vi "To Start and Stop (bare).vi"(4 "span":dbl, 6 "center":dbl) -> (0 "stop":dbl, 2 "start":dbl)   [LabVIEW 2017]
doc: "Takes two bare numbers that indicate the average (\"center\") and difference (\"span\") of two numbers and returns the beginning and end of the range."
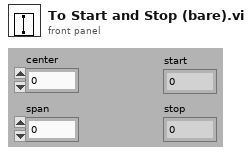
[diagram p1: front panel]
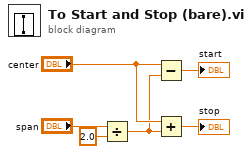
[diagram p0: block diagram]
diagram:
  n1 = Divide(x="span", y=2.0) -> (x/y=w3:dbl)
  n2 = Subtract(x="center", y=w3) -> (x-y=→"start":dbl)
  n3 = Add(x="center", y=w3) -> (x+y=→"stop":dbl)
